vi "CloseClean.vi"(8 "error in (no error)":errorcluster, 11 "hHandle":u32) -> (0 "error out":errorcluster)   [LabVIEW 2018, in "LibTiePie.lvlib"]
uses:
  LibTiePie.lvlib
  LabViewHS4/libtiepie.dll
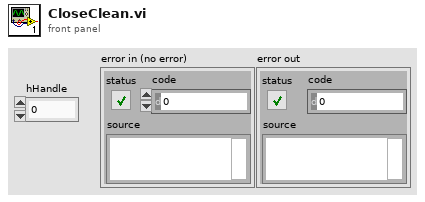
[diagram p1: front panel]
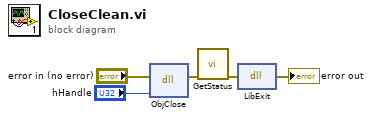
[diagram p0: block diagram]
diagram:
  n1 = dll-call lib="C:/Users/cwaha/Documents/LabViewHS4/libtiepie.dll" fn="ObjClose"(error in="error in (no error)", "hHandle"="hHandle") -> (error out=w2:errorcluster)  [unwired: 4 in, 1 out]
  n2 = call "GetStatus.vi"("error in (no error)"=w2) -> ("error out"=w5:errorcluster)  [unwired: 10 in]
  n3 = dll-call lib="C:/Users/cwaha/Documents/LabViewHS4/libtiepie.dll" fn="LibExit"(error in=w5) -> (error out=→"error out":errorcluster)  [unwired: 3 in, 1 out]
